vi "security_scanArguments.vi"(0 "ARGUMENTS":string[](array[string]), 1 "SCAN EXPRESSIONS":string[](array[string]), 2 "CHAR SEPARATOR":string, 4 "ENCRYPTION METHOD":u16(ring) items=["#0_none", "#1_hexa", "#2_hexa_scrambled"], 5 "ENCRYPTION FORMULA":string) -> (14 "PASSED ARGUMENTS":string[](array[string]))   [LabVIEW 2018, in "db_lib R3.lvlib"]
uses:
  db_lib R3.lvlib
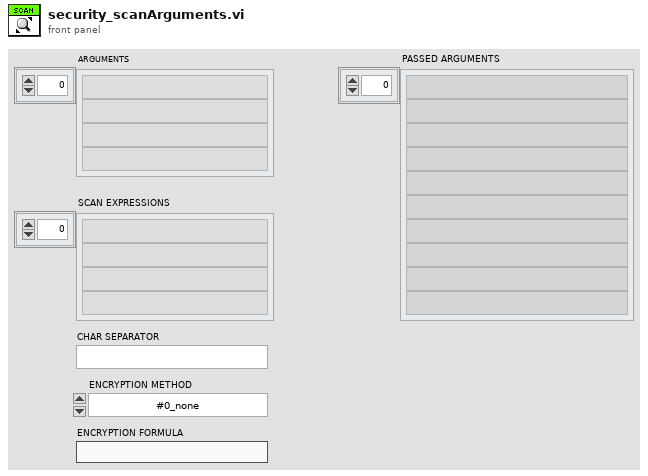
[diagram p1: front panel]
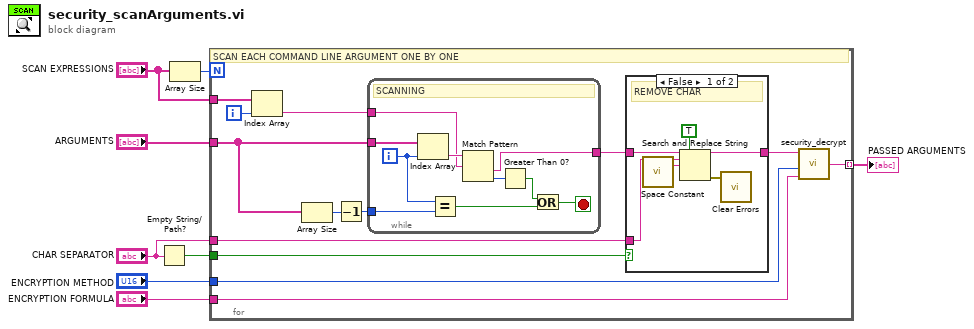
[diagram p0: block diagram]
diagram:
  n1 = Empty String/Path?(string/path="CHAR SEPARATOR") -> (empty?=w5:bool)
  n2 = Array Size(array="SCAN EXPRESSIONS") -> (size(s)=w8:i32)
  n3 = for {
    N: w8 -> [_]
    tunnel: "SCAN EXPRESSIONS" -> [w20]
    tunnel: "ARGUMENTS" -> [w19]
    tunnel: w5 -> [w15]
    tunnel: [w11] -> w3 mode=indexing
    tunnel: "CHAR SEPARATOR" -> [w13]
    tunnel: "ENCRYPTION METHOD" -> [w10]
    tunnel: "ENCRYPTION FORMULA" -> [w9]
    i -> [w21]
    # "SCAN EACH COMMAND LINE ARGUMENT ONE BY ONE"
    n4 = Index Array(array=w20, index=w21) -> (element=w18:string)
    n5 = Array Size(array=w19) -> (size(s)=w17:i32)
    n6 = Decrement(x=w17) -> (x-1=w16:i32)
    n7 = while {
      tunnel: w19 -> [w38]
      tunnel: w18 -> [w36]
      tunnel: w16 -> [w35]
      tunnel: [w29] -> w14
      i -> [w34]
      stop <- w30 stop-if-true
      # "SCANNING"
      n8 = Index Array(array=w38, index=w34) -> (element=w37:string)
      n9 = Equal?(x=w34, y=w35) -> (x = y?=w32:bool)
      n10 = Match Pattern(string=w37, regular expression=w36) -> (after substring=w29:string, offset past match=w33:i32)  [unwired: 1 in, 2 out]
      n11 = Greater Than 0?(x=w33) -> (x > 0?=w31:bool)
      n12 = Or(x=w31, y=w32) -> (x .or. y?=w30:bool)
    }
    n13 = case shown="False" w15 {
      tunnel: w14 -> [w27 w28]
      tunnel: [w24 w28] -> w12
      tunnel: w13 -> [w26 _]
      frame False {
        # "REMOVE CHAR"
        n14 = call <vilib>:"Space Constant.vi"() -> ("String"=w22:string)
        n15 = Search and Replace String(replace all?=TRUE ("replace all? (F)"), input string=w27, search string=w26, replace string=w22) -> (result string=w24:string, error out=w25:errorcluster)  [unwired: 4 in, 2 out]
        n16 = call <vilib>:"Clear Errors.vi"("error in (no error)"=w25) -> ()  [unwired: 5 in, 2 out]
      }
      frame True {
        # "DO NOTHING"
      }
    }
    n17 = call "security_decrypt.vi"("FORMULA (if any)"=w9, "METHOD"=w10, "ENCRYPTED DATA"=w12) -> ("RAW DATA"=w11:string)  [unwired: 3 in]
  }
  "PASSED ARGUMENTS" <- w3
